vi "toml_default_path.vi"() -> (1 "app file extension":string, 2 "app name":string, 3 "app.toml":path)   [LabVIEW 2017]
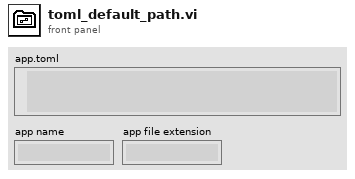
[diagram p1: front panel]
types:
  T1 = enum32{"invalid app kind", "Development System", "Run Time System", "Student Edition", "Embedded LabVIEW", "Evaluation", "Custom"}
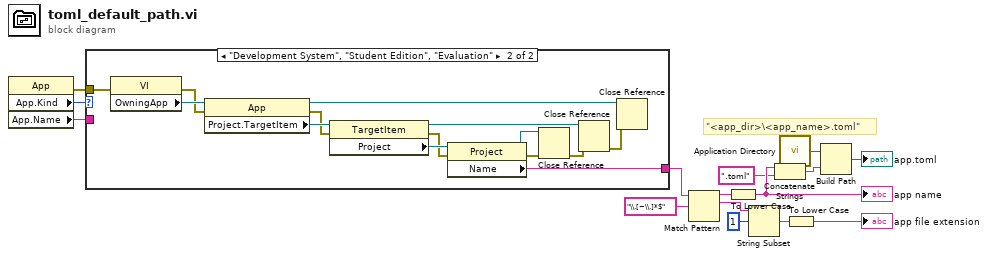
[diagram p0: block diagram]
diagram:
  # "\"<app_dir>\\<app_name>.toml\""
  n1 = property class="App"() -> (error out=w5:errorcluster, "App.Kind"=w8:T1, "App.Name"=w7:string)  [unwired: 2 in, 1 out]
  n2 = case shown="\"Development System\", \"Student Edition\", \"Evaluation\"" w8 {
    tunnel: w7 -> [w16 _]
    tunnel: [w16 w17] -> w6
    tunnel: w5 -> [_ w30]
    frame "invalid app kind", "Run Time System", "Embedded LabVIEW", "Custom" {
    }
    frame "Development System", "Student Edition", "Evaluation" {
      n3 = property class="VI"(error in=w30) -> (error out=w28:errorcluster, "OwningApp"=w29:refnum<vi>)  [unwired: 1 in, 1 out]
      n4 = property class="App"(reference=w29, error in=w28) -> (reference out=w19:refnum<vi>, error out=w26:errorcluster, "Project.TargetItem"=w27:refnum<vi>)
      n5 = property class="TargetItem"(reference=w27, error in=w26) -> (reference out=w21:refnum<vi>, error out=w24:errorcluster, "Project"=w25:refnum<vi>)
      n6 = property class="Project"(reference=w25, error in=w24) -> (reference out=w22:refnum<vi>, error out=w23:errorcluster, "Name"=w17:string)
      n7 = Close Reference(reference=w22, error in (no error)=w23) -> (error out=w20:errorcluster)
      n8 = Close Reference(reference=w21, error in (no error)=w20) -> (error out=w18:errorcluster)
      n9 = Close Reference(reference=w19, error in (no error)=w18) -> ()  [unwired: 1 out]
    }
  }
  n10 = Match Pattern(string=w6, regular expression="\\.[~\\.]*$") -> (before substring=w11:string, match substring=w4:string)  [unwired: 3 out]
  n11 = To Lower Case(string=w11) -> (all lower case string=w15:string)
  "app name" <- w15
  n12 = String Subset(string=w4, offset (0)=1) -> (substring=w2:string)  [unwired: 1 in]
  n13 = Concatenate Strings(w15, ".toml" ("string")) -> (w12:string)
  n14 = call <vilib>:"Application Directory.vi"() -> ("Application Directory"=w9:path)
  n15 = To Lower Case(string=w2) -> (all lower case string=→"app file extension":string)
  n16 = Build Path(base path=w9, name or relative path=w12) -> (appended path=→"app.toml":path)
